vi "MDAQ_TargetHelper.vi"(9 "Cluster IN":T1, 10 "XY Graph":refnum<vi>, 11 "Calibrated Graph":refnum<vi>) -> ()   [LabVIEW 2021]
uses:
  GUI_Def.ctl
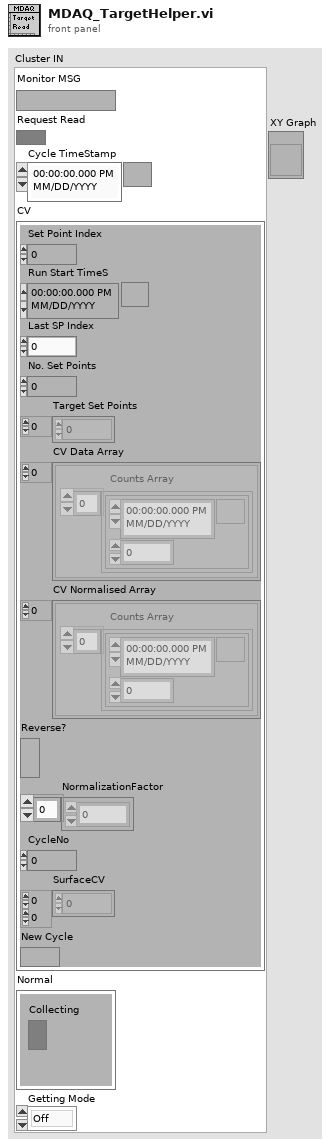
[diagram p1: front panel]
types:
  T1 = typedef "GUI_Def.ctl" = cluster{"Monitor MSG":string, "Request Read":bool, "Cycle TimeStamp":timestamp, "CV":cluster{"Set Point Index":u32, "Run Start TimeS":timestamp, "Last SP Index":u32, "No. Set Points":u32, "Target Set Points":dbl[], "CV Data Array":cluster{"Counts Array":cluster{timestamp, i32}[]}[], "CV Normalised Array":cluster{"Counts Array":cluster{timestamp, dbl}[]}[], "Reverse?":bool, "NormalizationFactor":i32[], "CycleNo":i32, "SurfaceCV":dbl[][], "New Cycle":bool}, "Normal":cluster{"Collecting":bool}, "Getting Mode":enum16{"Off", "Normal", "CV"}}
  T2 = cluster{"Name":string, "Color":u32, "Style":u8, "Point Style":u8, "Name Visible":bool, "Allow Drag":bool, "Cursor Mode":u32, "Plot":i32, "Index":i32, "Position":cluster{"X":dbl, "Y":dbl}, "X Scale":u32, "Y Scale":u32, "Watch Plots":i32[], "Watch All Plots":bool, "Plot Area":i32, "Label Offset":cluster{"X":dbl, "Y":dbl}}
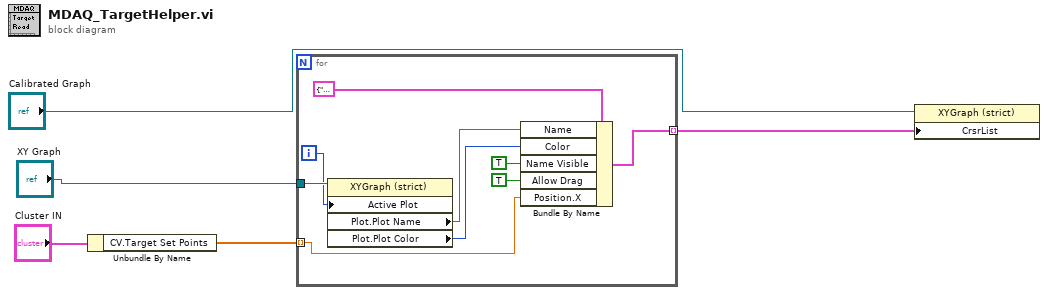
[diagram p0: block diagram]
diagram:
  n1 = Unbundle By Name("Cluster IN") -> ("CV.Target Set Points"=w4:dbl[])
  n2 = for {
    tunnel: w4 -> [w6] mode=indexing
    tunnel: [w13] -> w2 mode=indexing
    tunnel: "XY Graph" -> [w12]
    i -> [w11]
    n3 = property class="XYGraph (strict)"(reference=w12, "Active Plot"=w11) -> ("Plot.Plot Name"=w10:string, "Plot.Plot Color"=w9:u32)  [unwired: 1 in, 2 out]
    n4 = Bundle By Name(cluster=T2 {"Name"="", "Color"=0, "Style"=0, "Point Style"=0, "Name Visible"=FALSE, "Allow Drag"=FALSE, "Cursor Mode"=0, "Plot"=0, "Index"=0, "Position"={"X"=0.0, "Y"=0.0}, "X Scale"=0, "Y Scale"=0, "Watch Plots"=[], "Watch All Plots"=FALSE, "Plot Area"=0, "Label Offset"={"X"=0.0, "Y"=0.0}} ("element"), "Name"=w10, "Color"=w9, "Name Visible"=TRUE, "Allow Drag"=TRUE, "Position.X"=w6) -> (w13:T2)
  }
  n5 = property class="XYGraph (strict)"(reference="Calibrated Graph", "CrsrList"=w2) -> ()  [unwired: 1 in, 2 out]
